vi "Tell Child.vi"(4 "Priority":bool, 6 "UID":string, 7 "Actor in":refnum<class "Actor.lvclass">, 8 "Error in":errorcluster) -> (0 "Error out":errorcluster, 5 "Actor out":refnum<class "Actor.lvclass">)   [LabVIEW 2020, in "jettl.lvlib" / "Stopping jettl Msg.lvlib" / "Stopping.lvlib"]
doc: "jettl 6.12.1.94\nNathan Davis - Nathan Davis\nCopyright (c) 2026, Nathan Davis\nMIT"
uses:
  Stopping.lvlib
  Actor/Actor.lvclass
  jettl.lvlib
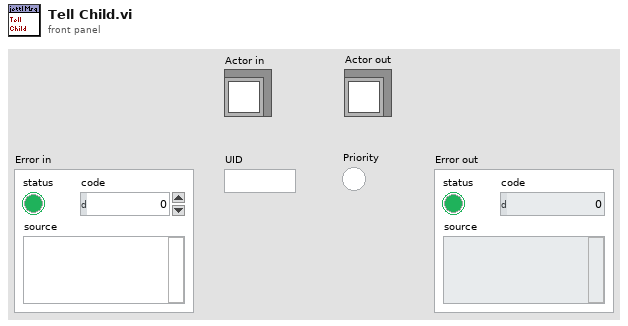
[diagram p1: front panel]
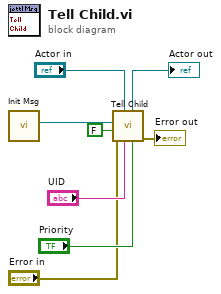
[diagram p0: block diagram]
diagram:
  n1 = call "Init Msg.vi"() -> ("Msg"=w1:refnum<class "Msg.lvclass">)  [unwired: 11 in]
  n2 = call "Tell Child.vi"("Priority"="Priority", "UID"="UID", "Actor in"="Actor in", "Error in"="Error in", "Reply"=FALSE, "Msg"=w1) -> ("Error out"=→"Error out":errorcluster, "Actor out"=→"Actor out":refnum<class "Actor.lvclass">)  [unwired: 4 in]
